vi "initialize-configuration.vi"(8 "error in (no error)":errorcluster, 11 "configuration":T1={"store_method"=enum."<store_method>", "rows"=-1, "columns"=-1}) -> (0 "error out":errorcluster, 3 "dvr":refnum<data-value>)   [LabVIEW 2015, in "lv-graph-global.lvlib"]
doc: "Initialize can be used to configure how much data can be stored and what happens when that max is reached. Use this to configure the expected number of rows, columns and the store method."
uses:
  _controls/configuration.ctl
  _controls/store_method.ctl
  _controls/data.ctl
  lv-graph-global.lvlib
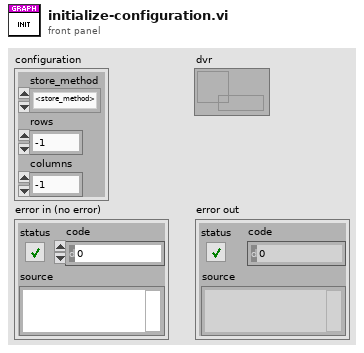
[diagram p1: front panel]
types:
  T1 = typedef "lv-graph-global.lvlib/configuration.ctl" = cluster{"store_method":T2, "rows":i32, "columns":i32}
  T2 = typedef "lv-graph-global.lvlib/store_method.ctl" = enum16{"<store_method>", "fixed", "grow"}
  T3 = typedef "lv-graph-global.lvlib/data.ctl" = cluster{"configuration":T1, "index":i32, "x_axis":dbl[], "y_axis":dbl[][]}
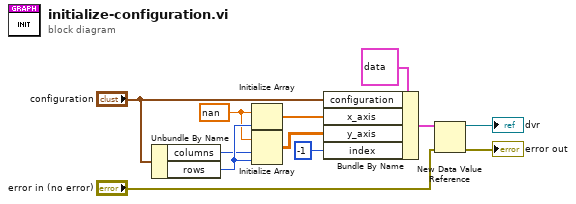
[diagram p0: block diagram]
diagram:
  w4 = nan
  n1 = Unbundle By Name("configuration") -> ("columns"=w8:i32, "rows"=w9:i32)
  n2 = Initialize Array(w4, w9) -> (w6:dbl[])
  n3 = Initialize Array(w4, w8, w9) -> (w7:dbl[][])
  n4 = Bundle By Name(cluster=T3 {"configuration"={"store_method"=enum."<store_method>", "rows"=-1, "columns"=-1}, "index"=0, "x_axis"=[], "y_axis"=[]} ("data"), "configuration"="configuration", "x_axis"=w6, "y_axis"=w7, "index"=-1 ("Index")) -> (w2:T3)
  n5 = New Data Value Reference(data value=w2, error in="error in (no error)") -> (data value reference=→"dvr":refnum<data-value>, error out=→"error out":errorcluster)
